vi "Execute 7z bat.vi"(8 "error in (no error)":errorcluster, 11 "PostBuildSupport in":refnum<class "PostBuildSupport (2013).lvclass">) -> (0 "error out":errorcluster, 3 "PostBuildSupport out":refnum<class "PostBuildSupport (2013).lvclass">)   [LabVIEW 2016, in "PostBuildSupport (2013).lvclass"]
uses:
  PostBuildSupport (2013).lvclass
  PostBuildSupport (2013).lvclass/PostBuildSupport (2013).ctl
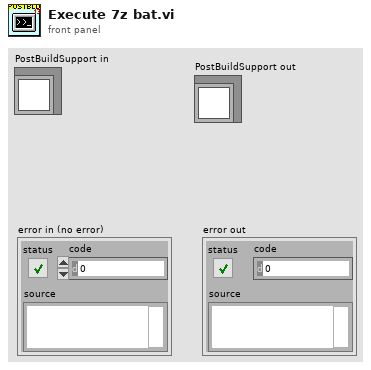
[diagram p1: front panel]
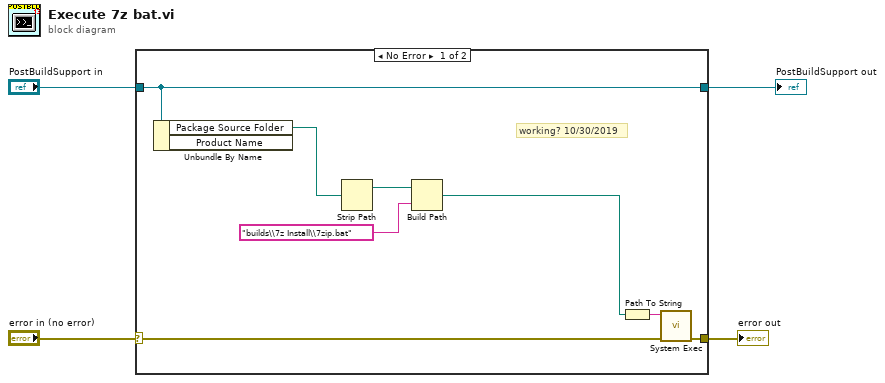
[diagram p0: block diagram]
diagram:
  n1 = case shown="No Error" "error in (no error)" {
    selector: "error in (no error)" -> [w8 w14]
    tunnel: [w12 w14] -> w1
    tunnel: "PostBuildSupport in" -> [w9 w13]
    tunnel: [w9 w13] -> w3
    frame No Error {
      # "working? 10/30/2019"
      n2 = Unbundle By Name(w9) -> ("Package Source Folder"=w11:path)  [unwired: 1 out]
      n3 = Strip Path(path=w11) -> (stripped path=w6:path)  [unwired: 1 out]
      n4 = Build Path(base path=w6, name or relative path="builds\\7z Install\\7zip.bat") -> (appended path=w5:path)
      n5 = Path To String(path=w5) -> (string=w7:string)
      n6 = call <vilib>:"System Exec.vi"("error in (no error)"=w8, "command line"=w7) -> ("error out"=w12:errorcluster)  [unwired: 6 in, 3 out]
    }
    frame Error {
    }
  }
  "error out" <- w1
  "PostBuildSupport out" <- w3
